vi "RSZVB Set RF Image Frequency.vi"(8 "error in (no error)":errorcluster {"code" format="%.0x"}, 9 "RF Image Frequency (Off)":bool, 10 "Channel (1)":i32=1, 11 "VISA session":refnum<visa-resource-name>) -> (0 "error out":errorcluster {"code" format="%.0x"}, 3 "dup VISA session":refnum<visa-resource-name>)   [LabVIEW 2011]
doc: "Prepares an additional mixer measurement at the second RF frequency (range) that the mixer converts to the selected IF frequency (RF Image Frequency). \n\nRemote-control command(s):\n[SENSe<Ch>:]FREQuency:CONVersion:MIXer:PRFimage"
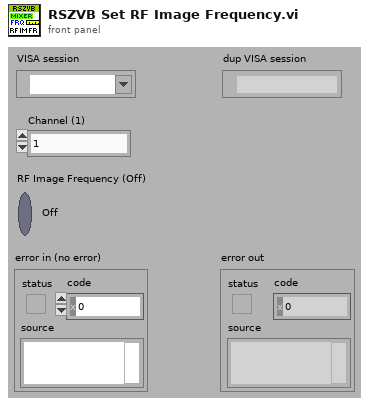
[diagram p1: front panel]
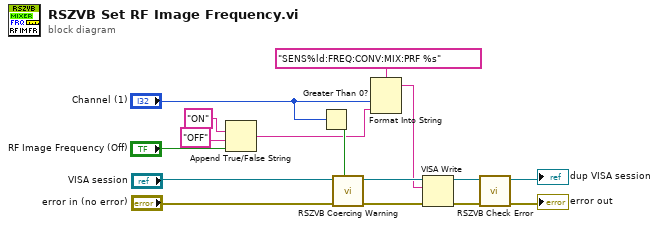
[diagram p0: block diagram]
diagram:
  n1 = Append True/False String(1:"RF Image Frequency (Off)", 2:"OFF", 3:"ON") -> (0:w1:string)  [unwired: 1 in]
  n2 = Greater Than 0?(x="Channel (1)") -> (x > 0?=w3:bool)
  n3 = call "RSZVB Coercing Warning.vi"("In Range?"=w3, "error in (no error)"="error in (no error)", "VISA session"="VISA session") -> ("error out"=w14:errorcluster, "dup VISA session"=w15:refnum<visa-resource-name>)  [unwired: 7 in]
  n4 = Format Into String(format string="SENS%ld:FREQ:CONV:MIX:PRF %s", "Channel (1)", w1) -> (resulting string=w11:string)  [unwired: 2 in, 1 out]
  n5 = VISA Write(VISA resource name=w15, write buffer=w11, error in (no error)=w14) -> (VISA resource name out=w12:refnum<visa-resource-name>, error out=w13:errorcluster)  [unwired: 1 out]
  n6 = call "RSZVB Check Error.vi"("error in (no error)"=w13, "VISA session"=w12) -> ("error out"=→"error out":errorcluster, "dup VISA session"=→"dup VISA session":refnum<visa-resource-name>)  [unwired: 8 in]
